vi "SetGenNOscNoise.vi"(3 "Enable Output":bool=TRUE, 5 "Input Voltage":dbl=1.0, 6 "Amp Scaler":dbl=1.0, 7 "NChannels":i32, 8 "error in (no error)":errorcluster, 9 "Output Voltage":dbl=1.0, 10 "Oscilloscope VISA":refnum<visa-resource-name>="Oscilloscope", 11 "Generator VISA":refnum<visa-resource-name>="Generator_1") -> (0 "error out 2":errorcluster)   [LabVIEW 2012]
uses:
  L0&L1/L0_BOARD_TESTs/trunk/Sum_Abrilader/L0_Sum_Adder Folder/C/Program Files/National Instruments/LabVIEW 2012/instr.lib/Agilent 81150/Agilent 81150.lvlib
  <instrlib>/Agilent 8000 Series/Agilent 8000 Series.lvlib
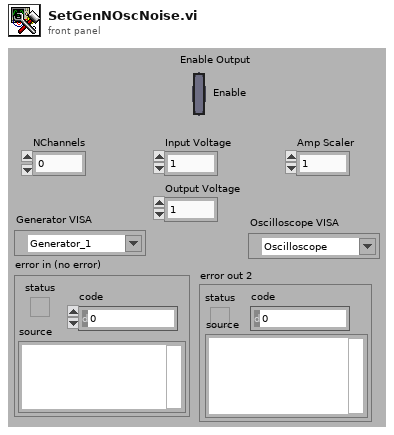
[diagram p1: front panel]
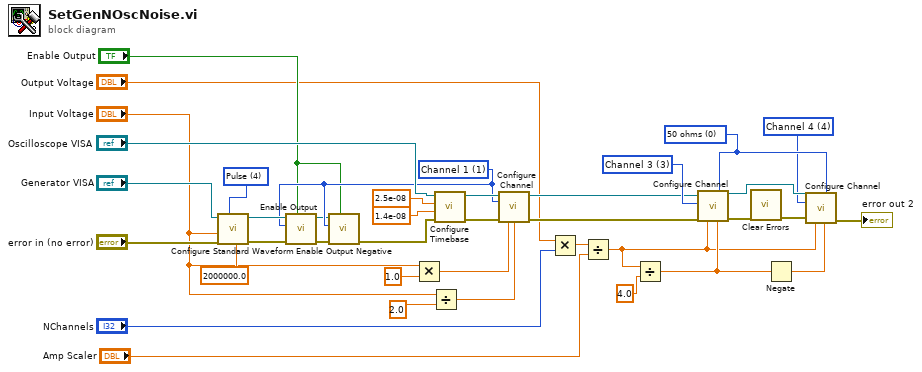
[diagram p0: block diagram]
diagram:
  w23 = u32 0 items=["50 ohms", "1 Mohms"] ("Input Impedance (1: 1 Mohms)")
  w21 = 3 items=["Channel 1"=1, "Channel 2"=2, "Channel 3"=3, "Channel 4"=4] ("Channel (1: Channel 1)")
  w20 = 4 items=["Channel 1"=1, "Channel 2"=2, "Channel 3"=3, "Channel 4"=4] ("Channel (1: Channel 1)")
  w7 = 1 items=["Channel 1"=1, "Channel 2"=2, "Channel 3"=3, "Channel 4"=4] ("Channel (1: Channel 1)")
  w38 = u16 4 items=["Sine", "Square", "Ramp Up", "Ramp Down", "Pulse", "Noise", "DC"] ("Waveform (0: Sine)")
  n1 = call <instrlib>:"Configure Standard Waveform.vi"("Frequency (1000.0 Hz)"=2000000.0, "Waveform (0: Sine)"=w38, "error in (no error)"="error in (no error)", "Amplitude (1.0 Vpp)"="Input Voltage", "VISA resource name"="Generator VISA") -> ("error out"=w9:errorcluster, "VISA resource name out"=w8:refnum<visa-resource-name>)  [unwired: 5 in]
  n2 = call <instrlib>:"Enable Output.vi"("Enable Output (T: Enable)"="Enable Output", "error in (no error)"=w9, "Channel (1: Channel1)"=w7, "VISA resource name"=w8) -> ("error out"=w5:errorcluster, "VISA resource name out"=w6:refnum<visa-resource-name>)  [unwired: 6 in]
  n3 = call "Enable Output Negative.vi"("Enable Output (T: Enable)"="Enable Output", "error in (no error)"=w5, "Channel (1: Channel1)"=w7, "VISA resource name"=w6) -> ("error out"=w4:errorcluster)  [unwired: 6 in, 1 out]
  n4 = Multiply(x="Input Voltage", y=1.0) -> (x*y=w32:dbl)
  n5 = Divide(x="Input Voltage", y=2.0) -> (x/y=w29:dbl)
  n6 = call "Configure Timebase.vi"("error in (no error)"=w4, "Position (0.0 s)"=1.4e-08, "Timebase (0.005 s)"=2.5e-08, "VISA resource name"="Oscilloscope VISA") -> ("error out"=w36:errorcluster, "VISA resource name out"=w35:refnum<visa-resource-name>)  [unwired: 6 in]
  n7 = call <instrlib>:"Configure Channel.vi"("VISA resource name"=w35, "Channel (1: Channel 1)"=w7, "error in (no error)"=w36, "Vertical Range (2.0 V)"=w32, "Vertical Offset (0.0 V)"=w29) -> ("VISA resource name out"=w15:refnum<visa-resource-name>, "error out"=w14:errorcluster)  [unwired: 9 in]
  n8 = Multiply(x="Output Voltage", y="NChannels") -> (x*y=w16:dbl)
  n9 = Divide(x=w16, y="Amp Scaler") -> (x/y=w1:dbl)
  n10 = Divide(x=w1, y=4.0) -> (x/y=w17:dbl)
  n11 = call <instrlib>:"Configure Channel.vi"("VISA resource name"=w15, "Input Impedance (1: 1 Mohms)"=w23, "Channel (1: Channel 1)"=w21, "error in (no error)"=w14, "Vertical Range (2.0 V)"=w1, "Vertical Offset (0.0 V)"=w17) -> ("VISA resource name out"=w24:refnum<visa-resource-name>, "error out"=w25:errorcluster)  [unwired: 8 in]
  n12 = call <vilib>:"Clear Errors.vi"("error in (no error)"=w25) -> ("error out"=w22:errorcluster)  [unwired: 6 in]
  n13 = Negate(x=w17) -> (-x=w19:dbl)
  n14 = call <instrlib>:"Configure Channel.vi"("VISA resource name"=w24, "Input Impedance (1: 1 Mohms)"=w23, "Channel (1: Channel 1)"=w20, "error in (no error)"=w22, "Vertical Range (2.0 V)"=w1, "Vertical Offset (0.0 V)"=w19) -> ("error out"=→"error out 2":errorcluster)  [unwired: 8 in, 1 out]
